vi "finder_switch.vi"(6 "error in":errorcluster, 7 "Micron config":T1, 8 "Finder":bool, 9 "Configuration":T4) -> (0 "error out":errorcluster)   [LabVIEW 2014]
uses:
  initialization/configuration.ctl
  initialization/asap_calibration.ctl
  <vilib>/Analysis/Matrix/Datatypes/RealMatrix.ctl
  micron/labview/initialization/micron_config.ctl
  micron/labview/manipulator/squiggle/Host/i2c_interface.ctl
  micron/labview/manipulator/squiggle/Host/fpga_reference.ctl
  micron/labview/testing/Micron params.ctl
  micron/labview/testing/stimulus.ctl
  micron/labview/testing/injection_point.ctl
  micron/labview/filtering/goal_loop_parms.ctl
  micron/labview/testing/mode_conrols.ctl
  micron/labview/testing/manipulator_cal.ctl
  testing/probe_calibration.ctl
  micron/labview/host/network_params.ctl
  micron/labview/cancellation/sq_control_params.ctl
  micron/labview/cancellation/decoupled_gain.ctl
  micron/labview/cancellation/estimation_controls.ctl
  initialization/globals.vi
  <vilib>/DAQmx/write.llb/DAQmx Write (Digital 1D Bool 1Chan 1Samp).vi
  <vilib>/Utility/error.llb/Error Cluster From Error Code.vi
  <vilib>/rvi/errors/niLvFpgaAdjustHostInterfaceError.vi
  <vilib>/rvi/interface/nirviReadWriteControl/nirviReadWriteControl.xnode
  micron/labview/manipulator/squiggle/FPGA Bitfiles/i2cmuxdemux.lvbitx
  NiFpgaLv.dll
  <vilib>/Analysis/Matrix/NI_Matrix.lvlib
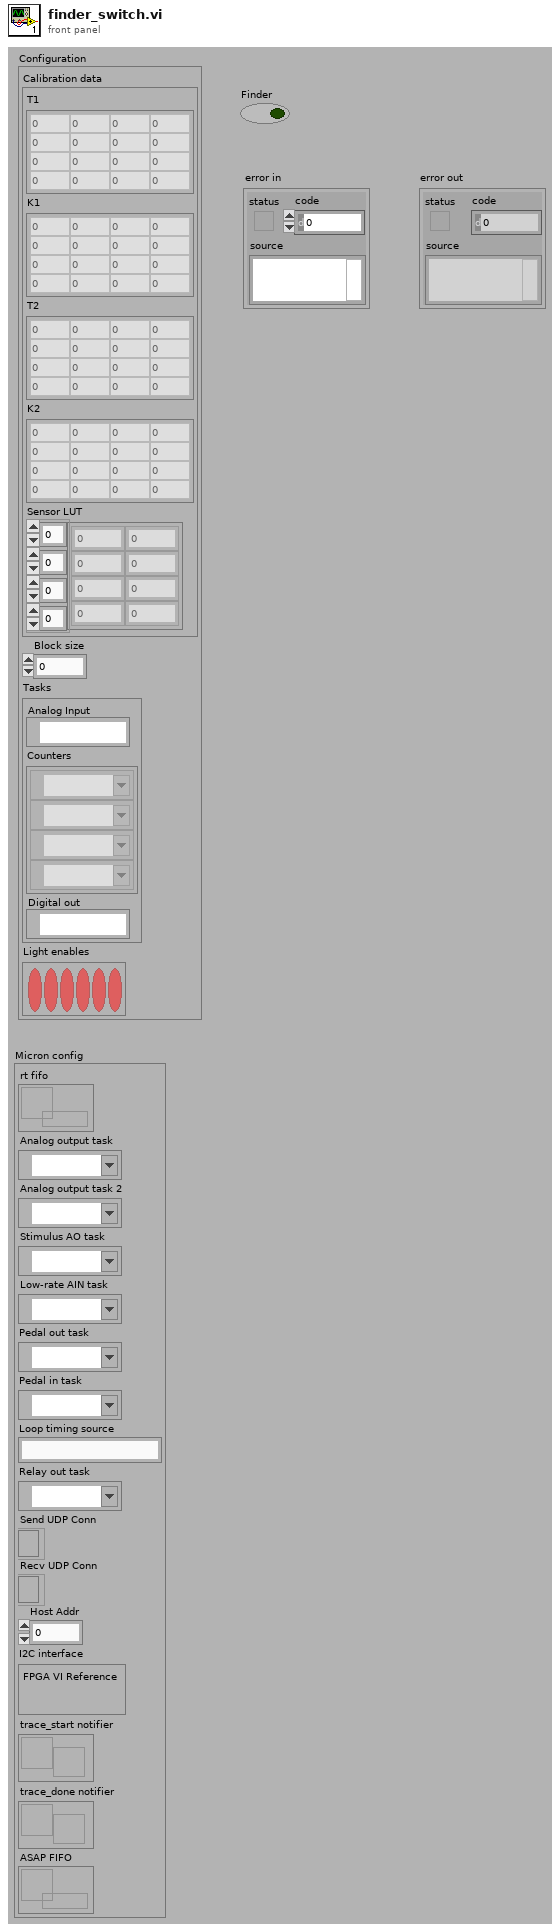
[diagram p1: front panel]
types:
  T1 = typedef "micron_config.ctl" = cluster{"rt fifo":refnum<k33>, "Analog output task":refnum<k21>, "Analog output task 2":refnum<k21>, "Stimulus AO task":refnum<k21>, "Low-rate AIN task":refnum<k21>, "Pedal out task":refnum<k21>, "Pedal in task":refnum<k21>, "Loop timing source":string, "Relay out task":refnum<k21>, "Send UDP Conn":refnum<k16>, "Recv UDP Conn":refnum<k16>, "Host Addr":u32, "I2C interface":T2, "trace_start notifier":refnum<notifier>, "trace_done notifier":refnum<notifier>, "ASAP FIFO":refnum<k33>}
  T2 = typedef "i2c_interface.ctl" = cluster{"FPGA VI Reference":T3}
  T3 = typedef "fpga_reference.ctl" = refnum<k20>
  T4 = typedef "configuration.ctl" = cluster{"Calibration data":T5, "Block size":i32, "Tasks":cluster{"Analog Input":refnum<k21>, "Counters":refnum<k21>[], "Digital out":refnum<k21>}, "Light enables":bool[]}
  T5 = typedef "asap_calibration.ctl" = cluster{"T1":T6, "K1":T6, "T2":T6, "K2":T6, "Sensor LUT":sgl[][][][]}
  T6 = typedef "NI_Matrix.lvlib/RealMatrix.ctl" = dbl[][]
  T7 = enum16{"ASAP/Trigger", "ASAP/Finder", "ASAP/Micron", "ASAP/Micron 2", "Micron 6DOF"}
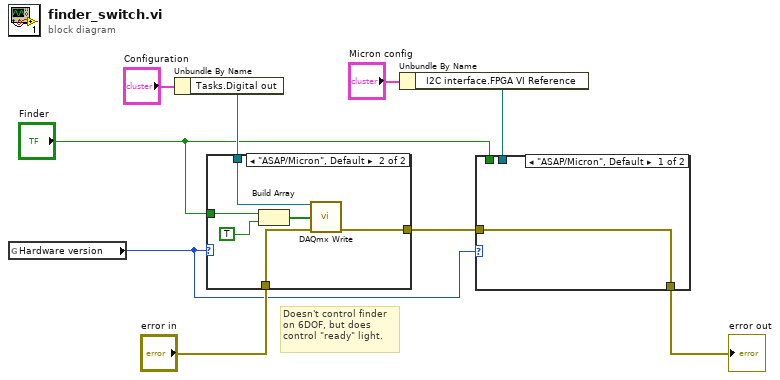
[diagram p0: block diagram]
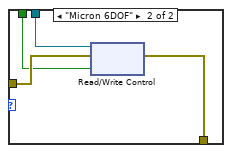
[diagram p2: hidden frame]
diagram:
  # "Doesn't control finder\non 6DOF, but does \ncontrol \"ready\" light."
  n1 = global read "globals.vi" "Hardware version"() -> (w5:T7)
  n2 = Unbundle By Name("Configuration") -> ("Tasks.Digital out"=w8:refnum<k21>)
  n3 = case shown="\"ASAP/Micron\", Default" w5 {
    tunnel: "Finder" -> [_ w15]
    tunnel: w8 -> [_ w13]
    tunnel: "error in" -> [w10 w12]
    tunnel: [w10 w11] -> w4
    frame "ASAP/Trigger" {
    }
    frame "ASAP/Micron", Default {
      n4 = Build Array(w15, TRUE ("element")) -> (w14:bool[])
      n5 = call-poly <vilib>:"DAQmx Write.vi"("task/channels in"=w13, "data"=w14, "error in"=w12) -> ("error out"=w11:errorcluster)  [unwired: 1 in, 11 out]
    }
  }
  n6 = Unbundle By Name("Micron config") -> ("I2C interface.FPGA VI Reference"=w3:T3)
  n7 = case shown="\"ASAP/Micron\", Default" w5 {
    tunnel: [w17 w21] -> w1
    tunnel: w4 -> [w17 w20]
    tunnel: w3 -> [_ w19]
    tunnel: "Finder" -> [_ w18]
    frame "ASAP/Micron", Default {
    }
    frame "Micron 6DOF" {
      n8 = xnode "Read/Write Control"("FPGA VI Reference In"=w19, "error in"=w20, "Finder"=w18) -> ("error out"=w21:errorcluster)  [unwired: 1 out]
    }
  }
  "error out" <- w1
